vi "Get Digest.vi"(11 "Hash Function in":refnum<class "NI_SHA-256.lvclass">) -> (2 "Digest":u8[](array[numeric]) format="%02x", 3 "Hash Function out":refnum<class "NI_SHA-256.lvclass">)   [LabVIEW 2013, in "NI_SHA-256(2013).lvlib" / "NI_SHA-256.lvclass"]
doc: "Compute the message digest given previously supplied input blocks."
uses:
  NI_SHA-256.lvclass
  NI_SHA-256.lvclass/NI_SHA-256.ctl
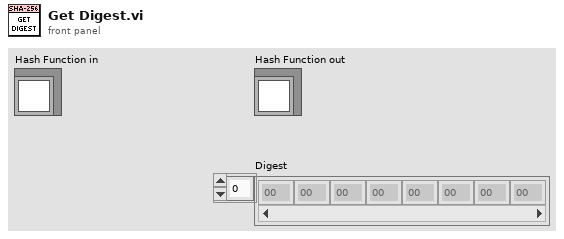
[diagram p1: front panel]
types:
  T1 = typedef "NI_SHA-256(2013).lvlib/NI_SHA-256.lvclass/Mode.ctl" = enum16{"SHA-256", "SHA-224"}
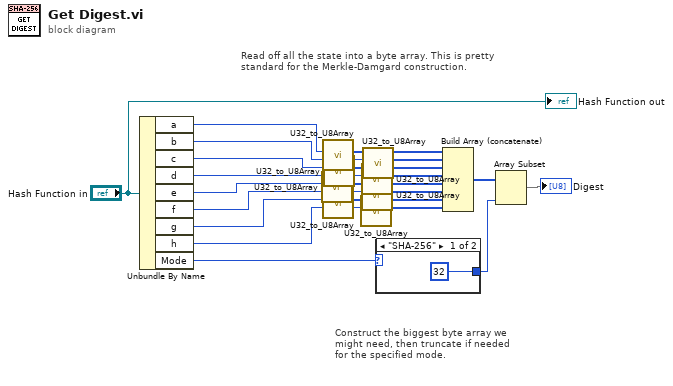
[diagram p0: block diagram]
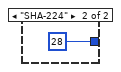
[diagram p2: hidden frame]
diagram:
  # "Construct the biggest byte array we might need, then truncate if needed for the specified mode."
  # "Read off all the state into a byte array. This is pretty standard for the Merkle-Damgard construction."
  n1 = Unbundle By Name("Hash Function in") -> ("a"=w16:u32, "b"=w14:u32, "c"=w13:u32, "d"=w10:u32, "e"=w4:u32, "f"=w3:u32, "g"=w2:u32, "h"=w1:u32, "Mode"=w19:T1)
  n2 = call "U32_to_U8Array.vi"("U32"=w4) -> ("U8"=w8:u8[])  [unwired: 10 in]
  n3 = call "U32_to_U8Array.vi"("U32"=w16) -> ("U8"=w15:u8[])  [unwired: 10 in]
  n4 = call "U32_to_U8Array.vi"("U32"=w2) -> ("U8"=w6:u8[])  [unwired: 10 in]
  n5 = call "U32_to_U8Array.vi"("U32"=w13) -> ("U8"=w11:u8[])  [unwired: 10 in]
  n6 = call "U32_to_U8Array.vi"("U32"=w1) -> ("U8"=w5:u8[])  [unwired: 10 in]
  n7 = call "U32_to_U8Array.vi"("U32"=w10) -> ("U8"=w9:u8[])  [unwired: 10 in]
  n8 = call "U32_to_U8Array.vi"("U32"=w3) -> ("U8"=w7:u8[])  [unwired: 10 in]
  n9 = call "U32_to_U8Array.vi"("U32"=w14) -> ("U8"=w12:u8[])  [unwired: 10 in]
  n10 = case shown="\"SHA-256\"" w19 {
    tunnel: [32 28] -> w18
    frame "SHA-256" {
    }
    frame "SHA-224" {
    }
  }
  n11 = Build Array (concatenate)(w15, w12, w11, w9, w8, w7, w6, w5) -> (w20:u8[])
  n12 = Array Subset(array=w20, length=w18) -> (→"Digest":u8[])  [unwired: 1 in]
  "Hash Function out" <- "Hash Function in"
